vi "Cascade.vi"(0 "LV MDI in":refnum<class "LV MDI.lvclass">, 5 "Order":u16(ring), 11 "error in (no error)":errorcluster) -> (4 "LV MDI out":refnum<class "LV MDI.lvclass">, 15 "error out":errorcluster)   [LabVIEW 2016, in "LV MDI.lvclass"]
uses:
  LV MDI.lvclass
  LV MDI.lvclass/LV MDI.ctl
  user32.dll
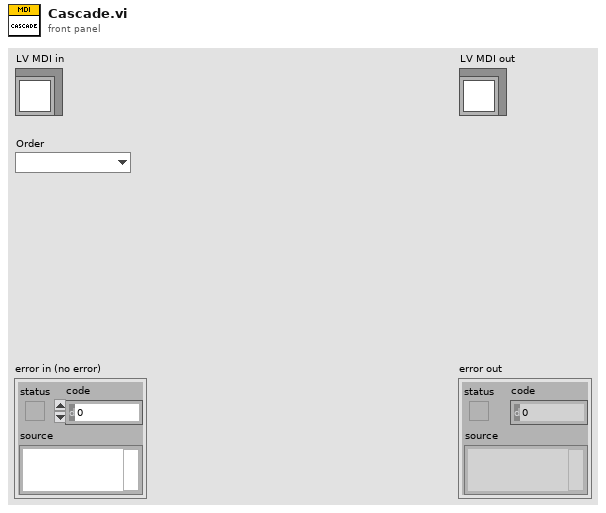
[diagram p1: front panel]
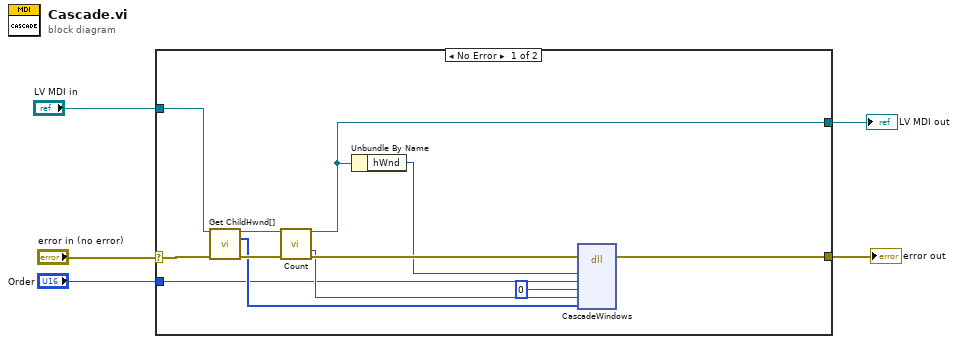
[diagram p0: block diagram]
diagram:
  n1 = case shown="No Error" "error in (no error)" {
    selector: "error in (no error)" -> [w15 w19]
    tunnel: [w10 w19] -> w4
    tunnel: [w13 w18] -> w2
    tunnel: "LV MDI in" -> [w14 w18]
    tunnel: "Order" -> [w6 _]
    frame No Error {
      n2 = call "Get ChildHwnd[].vi"("LV MDI in"=w14, "error in (no error)"=w15) -> ("LV MDI out"=w16:refnum<class "LV MDI.lvclass">, "ChildHwnd[]"=w7:u32[], "error out"=w17:errorcluster)  [unwired: 11 in]
      n3 = call "Count.vi"("LV MDI in"=w16, "error in (no error)"=w17) -> ("LV MDI out"=w13:refnum<class "LV MDI.lvclass">, "Count"=w8:i32, "error out"=w11:errorcluster)  [unwired: 11 in]
      n4 = Unbundle By Name(w13) -> ("hWnd"=w9:i32)
      n5 = dll-call lib="user32.dll" fn="CascadeWindows"(error in=w11, "hwndParent"=w9, "wHow"=w6, "lpRect"=0 ("wHow"), "cKids"=w8, "lpKids"=w7) -> (error out=w10:errorcluster)  [unwired: 8 in, 1 out]
    }
    frame Error {
    }
  }
  "error out" <- w4
  "LV MDI out" <- w2
